vi "GetSingleMeasurementValues.vi"(8 "Error in":errorcluster, 11 "DevicesAndSignals":T1) -> (0 "Error out":errorcluster, 1 "MeasurementValues(Waveform)":waveform(dbl)[](array[waveform]), 3 "DevicesAndSignals":T1)   [LabVIEW 2016]
doc: "Obtains one single measurement value for each given signal without initializing a continuous measurement. Filter settings will be ignored."
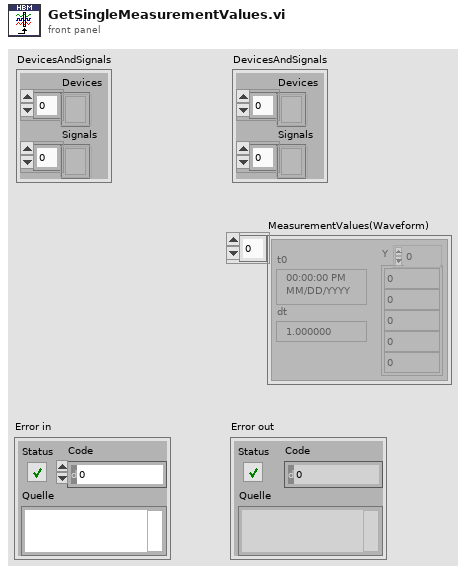
[diagram p1: front panel]
types:
  T1 = cluster{"Devices":refnum<k24>[], "Signals":refnum<k24>[]}
  T2 = typedef "LVDateTimeRec.ctl" = cluster{"Sekundenbruchteil":dbl, "Sekunde":i32, "Minute":i32, "Stunde":i32, "Tag des Monats":i32, "Monat":i32, "Jahr":i32, "Wochentag":i32, "Tag des Jahres":i32, "DST":i32}
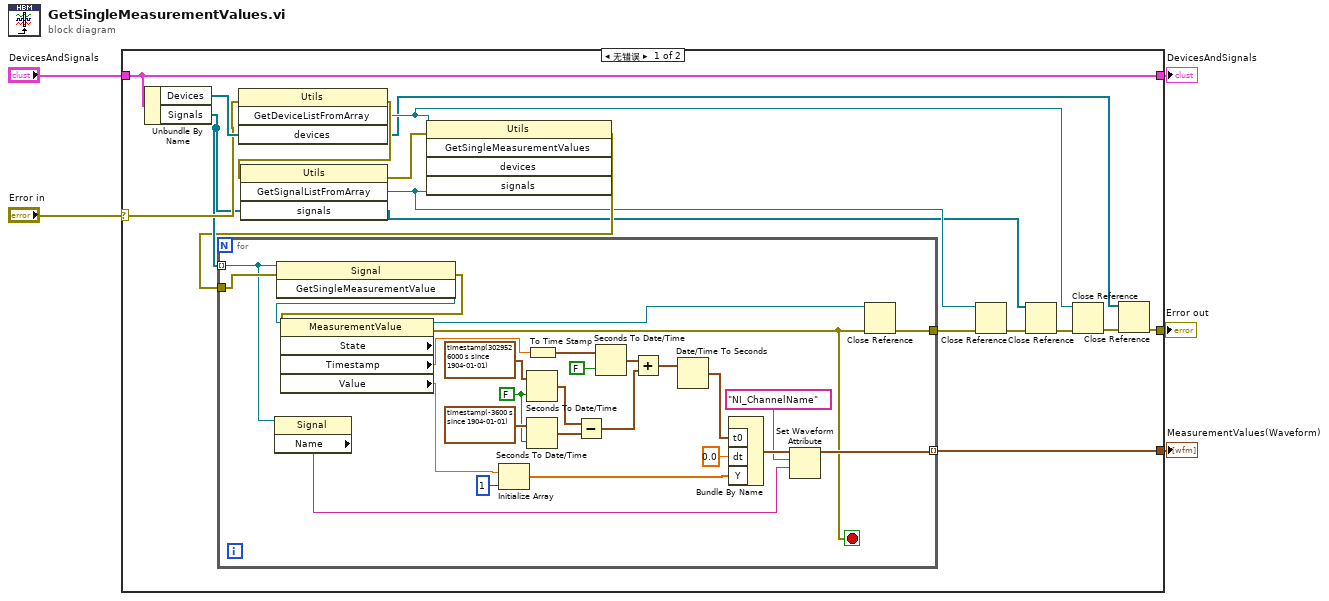
[diagram p0: block diagram]
diagram:
  n1 = case shown="无错误" "Error in" {
    selector: "Error in" -> [w20 w51]
    tunnel: "DevicesAndSignals" -> [w22 w50]
    tunnel: [w8 w51] -> w3
    tunnel: [w22 w50] -> w2
    tunnel: [w15 _] -> w1
    frame No Error {
      n2 = Unbundle By Name(w22) -> ("Devices"=w21:refnum<k24>[], "Signals"=w17:refnum<k24>[])
      n3 = invoke on="Methodenknoten" class="Utils" method="GetDeviceListFromArray"(error in=w20, "devices"=w21) -> (error out=w18:errorcluster, "GetDeviceListFromArray"=w10:refnum<k24>, "devices"=w6:refnum<k24>[])  [unwired: 2 in, 1 out]
      n4 = invoke on="Methodenknoten" class="Utils" method="GetSignalListFromArray"(error in=w18, "signals"=w17) -> (error out=w19:errorcluster, "GetSignalListFromArray"=w13:refnum<k24>, "signals"=w9:refnum<k24>[])  [unwired: 2 in, 1 out]
      n5 = invoke on="Methodenknoten" class="Utils" method="GetSingleMeasurementValues"(error in=w19, "devices"=w10, "signals"=w13) -> (error out=w16:errorcluster)  [unwired: 2 in, 4 out]
      n6 = for {
        tunnel: w17 -> [w30] mode=indexing
        tunnel: w16 -> [w48]
        tunnel: [w28] -> w15 mode=indexing
        tunnel: [w25] -> w14
        stop <- w24 stop-if-true
        w44 = FALSE ("in Weltzeit (F)")
        n7 = property on="Eigenschaftsknoten" class="Signal"(reference=w30) -> ("Name"=w27:string)  [unwired: 1 in, 2 out]
        n8 = invoke on="Methodenknoten" class="Signal" method="GetSingleMeasurementValue"(reference=w30, error in=w48) -> (error out=w47:errorcluster, "GetSingleMeasurementValue"=w49:refnum<k24>)  [unwired: 1 in, 1 out]
        n9 = property on="Eigenschaftsknoten" class="MeasurementValue" props=["State", "Timestamp", "Value"](reference=w49, error in=w47) -> (reference out=w23:refnum<k24>, error out=w24:errorcluster, "Timestamp"=w34:dbl, "Value"=w33:dbl)  [unwired: 1 out]
        n10 = Initialize Array(w33, 1 ("Dimension")) -> (w31:dbl[])
        n11 = Seconds To Date/Time(time stamp (now)=timestamp(3029526000 s since 1904-01-01), to UTC (F)=w44) -> (date time rec=w37:T2)
        n12 = Seconds To Date/Time(time stamp (now)=timestamp(-3600 s since 1904-01-01), to UTC (F)=w44) -> (date time rec=w38:T2)
        n13 = To Time Stamp(1:w34) -> (0:w43:timestamp)
        n14 = Subtract(x=w37, y=w38) -> (x-y=w41:T2)
        n15 = Seconds To Date/Time(time stamp (now)=w43, to UTC (F)=FALSE ("in Weltzeit (F)")) -> (date time rec=w42:T2)
        n16 = Add(x=w42, y=w41) -> (x+y=w40:T2)
        n17 = Date/Time To Seconds(2:w40) -> (0:w29:timestamp)  [unwired: 1 in]
        n18 = Bundle By Name("t0"=w29, "dt"=0.0, "Y"=w31) -> (w36:waveform(dbl))  [unwired: 1 in]
        n19 = Set Waveform Attribute(5:w27, 6:"NI_ChannelName" ("Channel Name"), 7:w36) -> (3:w28:waveform(dbl))  [unwired: 1 in, 2 out]
        n20 = Close Reference(reference=w23, error in (no error)=w24) -> (error out=w25:errorcluster)
      }
      n21 = Close Reference(reference=w13, error in (no error)=w14) -> (error out=w12:errorcluster)
      n22 = Close Reference(reference=w9, error in (no error)=w12) -> (error out=w11:errorcluster)
      n23 = Close Reference(reference=w10, error in (no error)=w11) -> (error out=w7:errorcluster)
      n24 = Close Reference(reference=w6, error in (no error)=w7) -> (error out=w8:errorcluster)
    }
    frame Error {
    }
  }
  "Error out" <- w3
  "DevicesAndSignals" <- w2
  "MeasurementValues(Waveform)" <- w1
